vi "Mono Sample API.vi"() -> ()   [LabVIEW 2021]
uses:
  Controls/Data highway.ctl
  Controls/LED intensity Command.ctl
  Controls/State Comm.ctl
  Controls/API Command.ctl
  5323141f-2985-4b05-94d1-ece9b0648710.vi
  4ae9b108-370e-49ae-8d4b-02a5277f3aaa.vi
  <vilib>/Instr/_visa.llb/VISA Configure Serial Port (Instr).vi
panel:
  in  "offset":dbl
  in  "Comm":T1=enum."Grating Density@1"
  in  "Filter Num":i32
  in  "Refresh Button":bool
  in  "Intensity Value":i32
  out "Intensity?":bool
  in  "Intensity":bool
  out "Grating":bool
  out "Device check":bool
  in  "Device Check":bool
  in  "Set GRating Density":bool
  out "Connection?":bool
  out "error out 2":errorcluster
  out "Port out":refnum<visa-resource-name>
  out "Final response":u8
  in  "Slit":string
  out "Response":u8
  in  "error in":errorcluster
  in  "Port":refnum<visa-resource-name>
  out "Connected?":bool
  out "result":bool
  out "State":T2
  out "Wavelength":bool
  out "Shutter":bool
  out "filter":bool
  in  "Filter":bool
  in  "Shutter":bool
  in  "Wavelength(nm)":i32 min=100
  in  "Stop":bool
  out "Array":bool[](array[boolean])
  out "error out":errorcluster
  in  "error in (no error)":errorcluster
  in  "Data in out":T3={"MonoCr Port"="COM3", "Grating Selection"=enum."Grating@1", "Connection?"=TRUE, "LED Comm"=enum."LED@1", "Intensity Value"=20, "Grating Number"=1, "Wavenumber"=0, "Slit Width"=8, "Filter Num"=3, "Grating Density"=1200, "Wavelength(nm)"=532, "offset"=0.0}
  in  "Set wavelength":bool
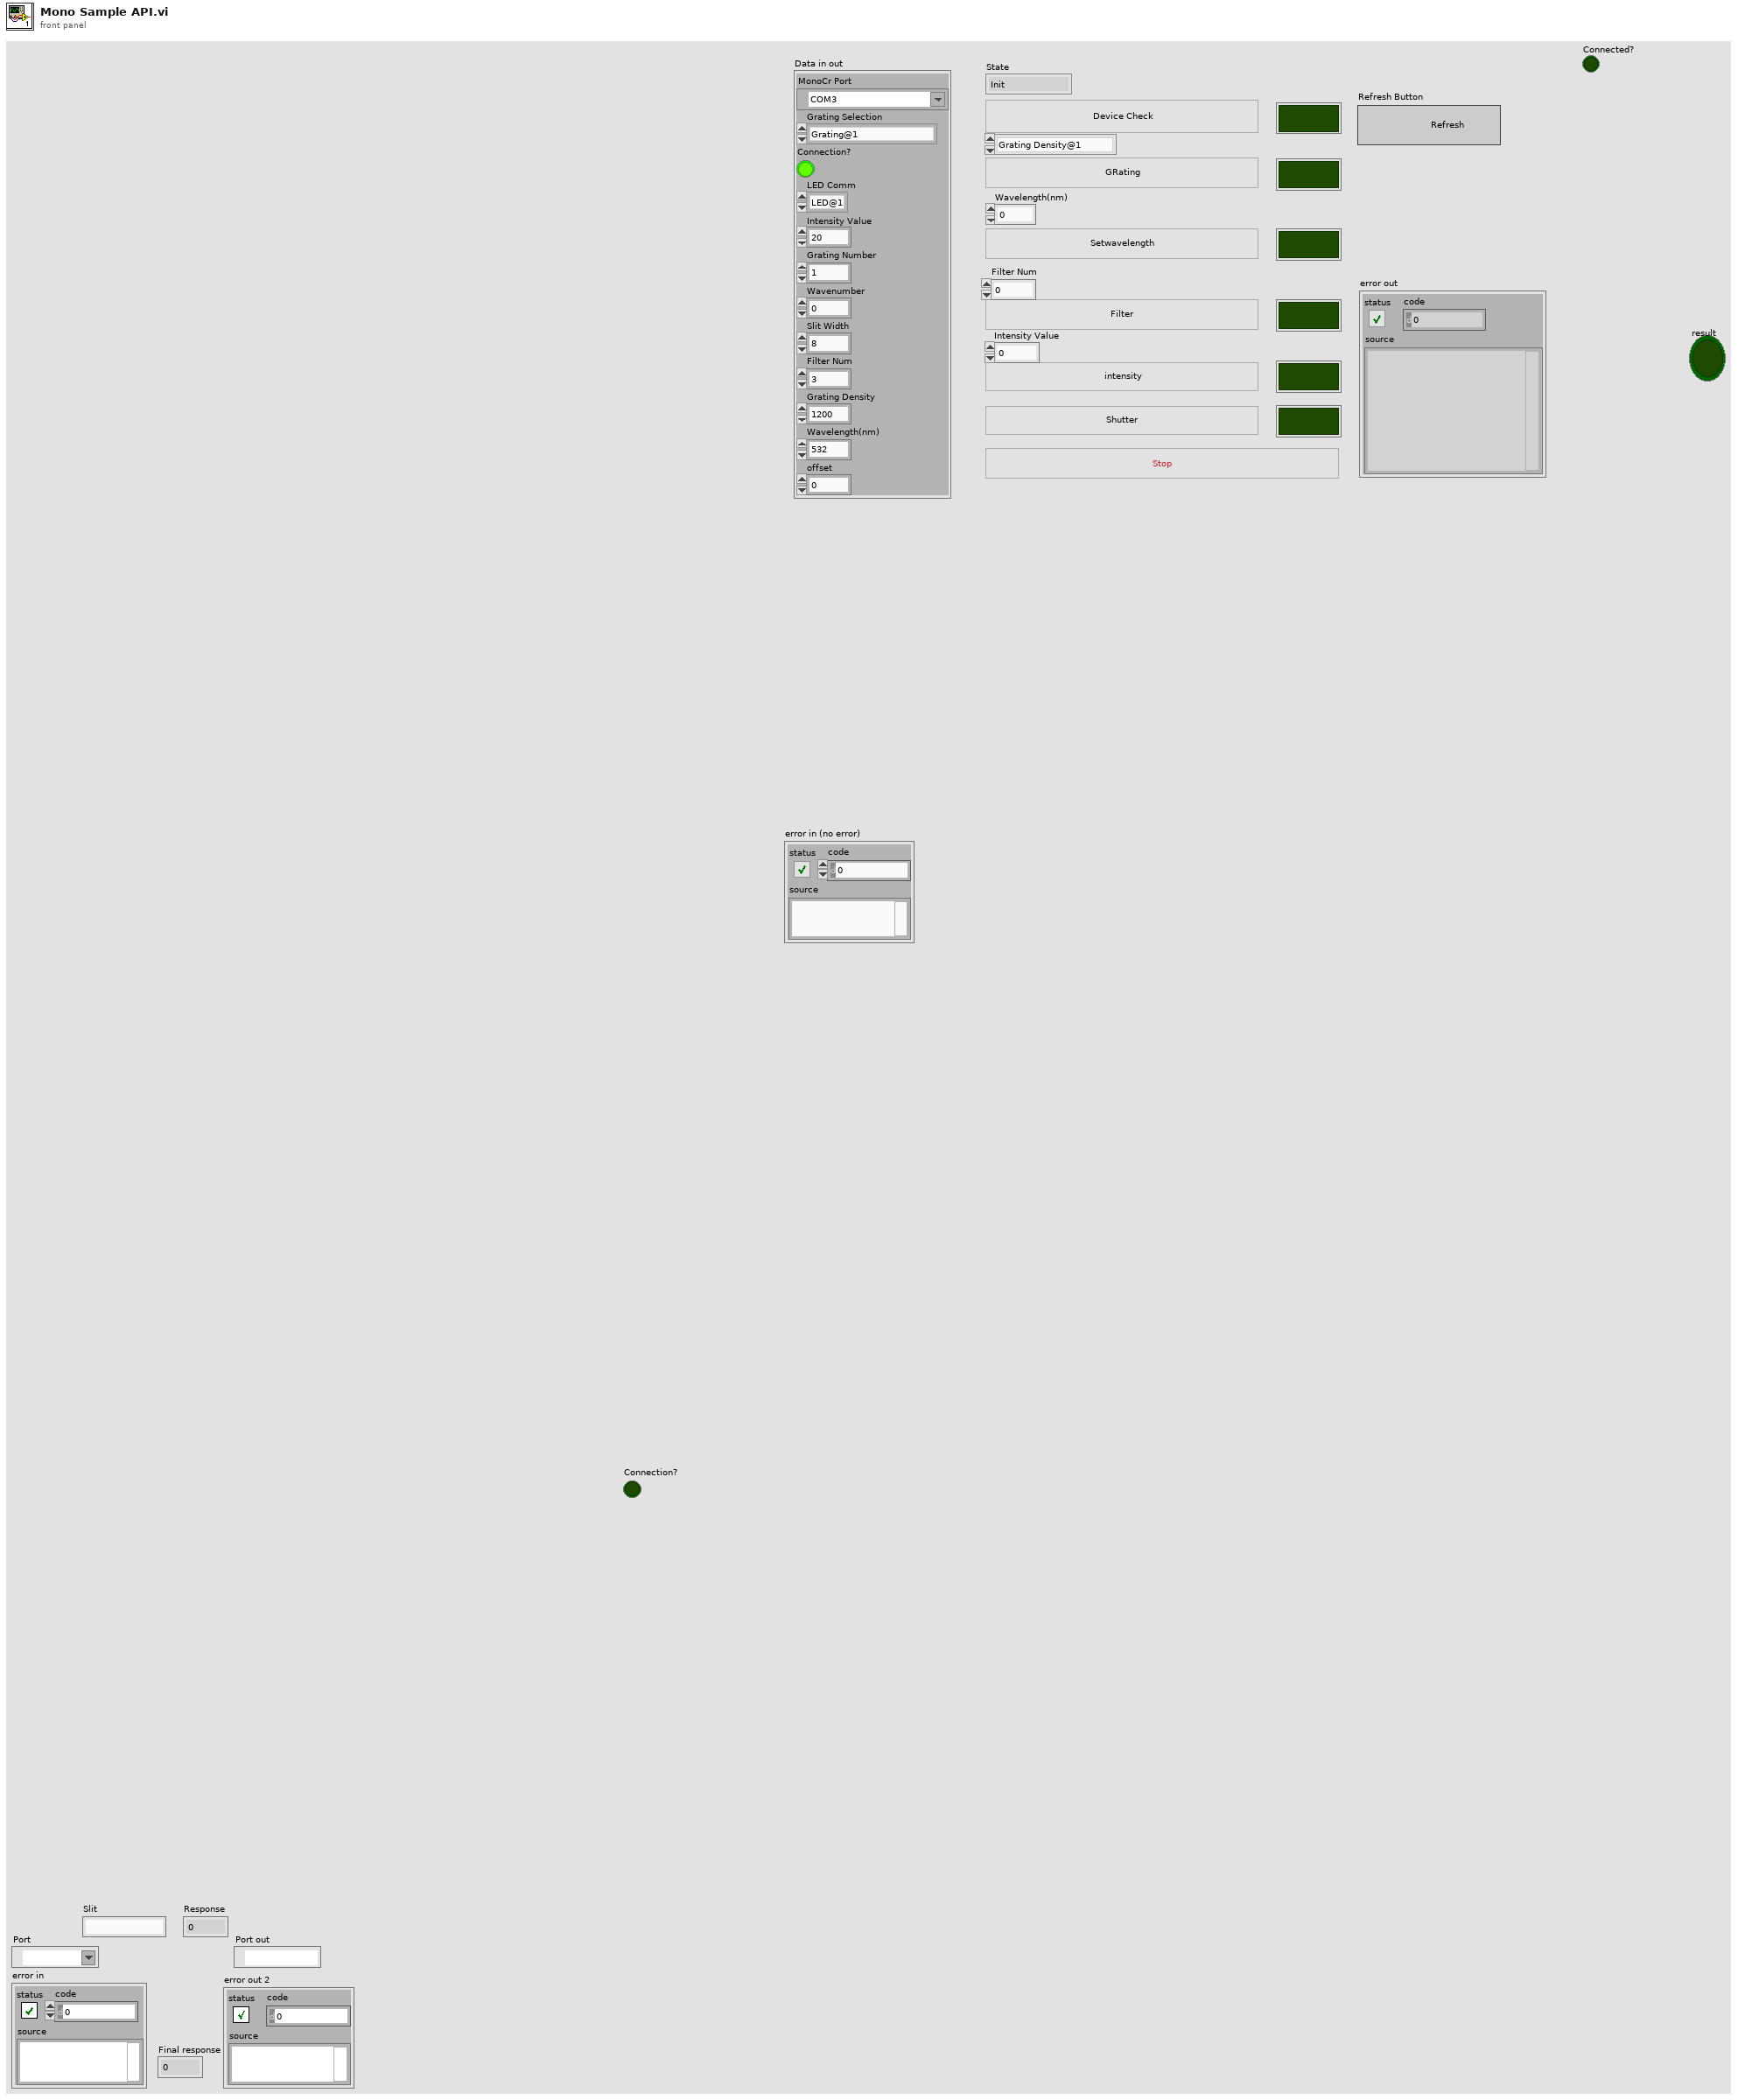
[diagram p1: front panel]
types:
  T1 = typedef "API Command.ctl" = enum16{"Init", "Device Check", "Grating Density@1", "Grating Density@2", "SetWavelength", "Filter Selection", "Shutter open", "Shutter close", "LED Intensity", "Set Grating", "Slit Width", "Stop running", "Reset Mono", "Close"}
  T2 = typedef "State Comm.ctl" = enum16{"Init", "Main", "Close"}
  T3 = typedef "Data highway.ctl" = cluster{"MonoCr Port":refnum<visa-resource-name>, "Grating Selection":enum16{"Grating@1", "Grating@2"}, "Connection?":bool, "LED Comm":T4, "Intensity Value":i32, "Grating Number":i32, "Wavenumber":i32, "Slit Width":i32, "Filter Num":i32, "Grating Density":i32, "Wavelength(nm)":i32, "offset":dbl}
  T4 = typedef "LED intensity Command.ctl" = enum16{"LED@1", "LED@2"}
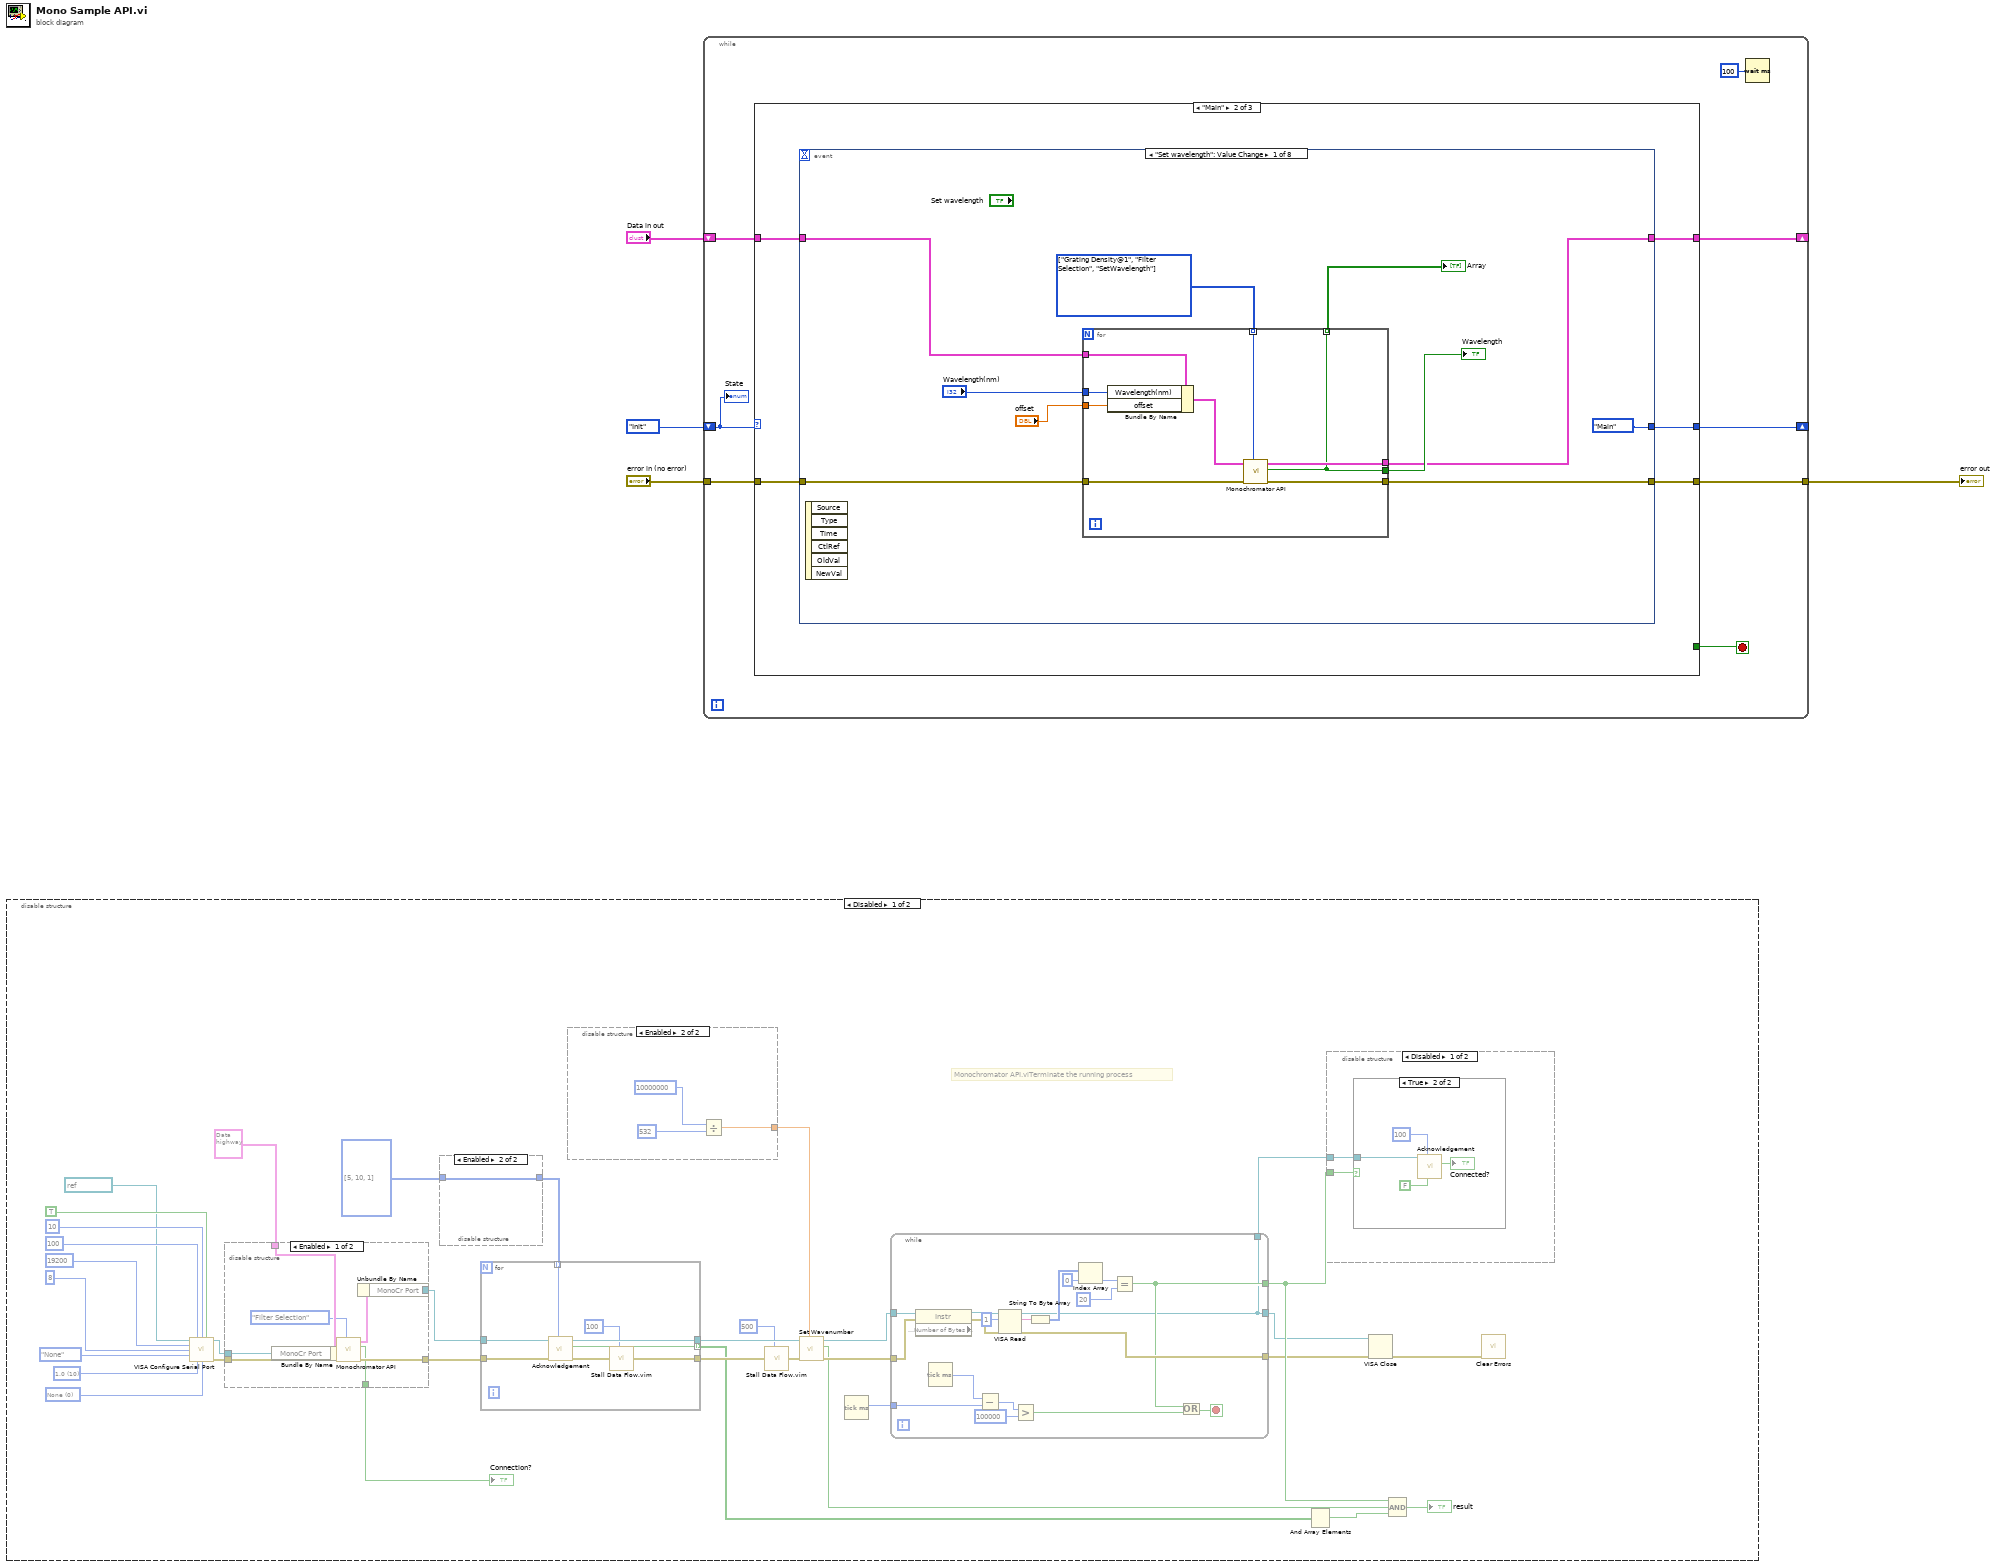
[diagram p0: block diagram]
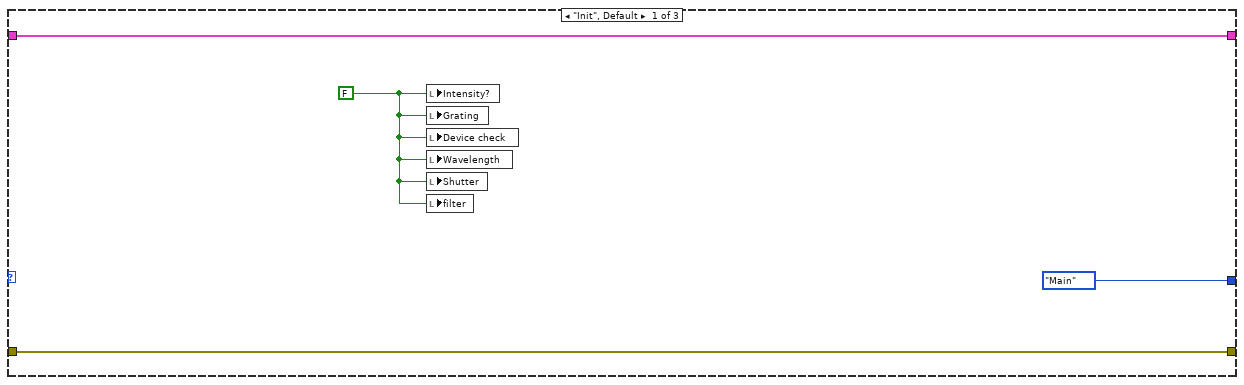
[diagram p2: hidden frame]
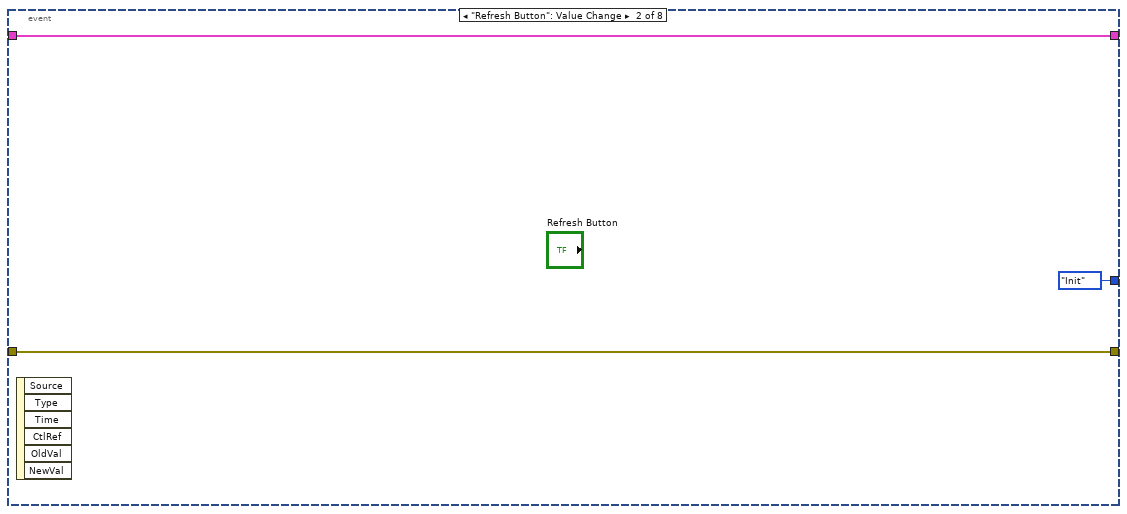
[diagram p3: hidden frame]
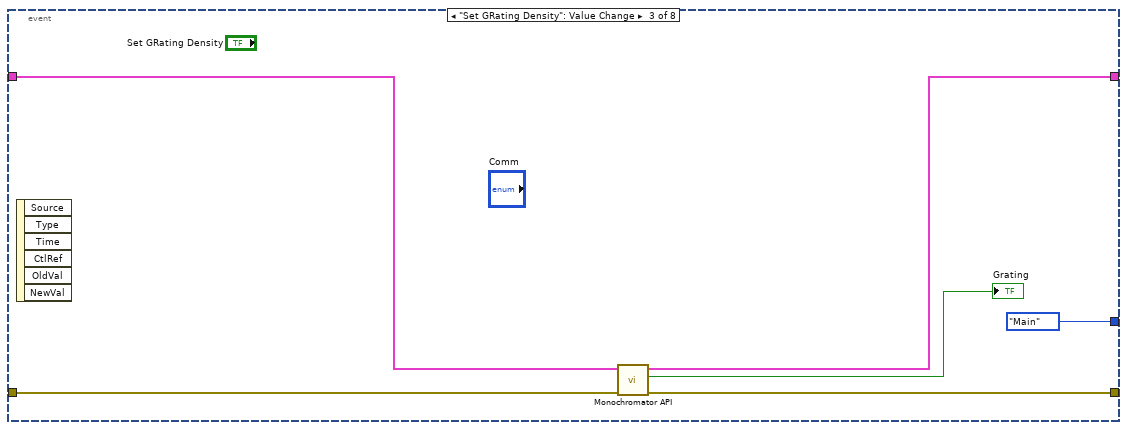
[diagram p4: hidden frame]
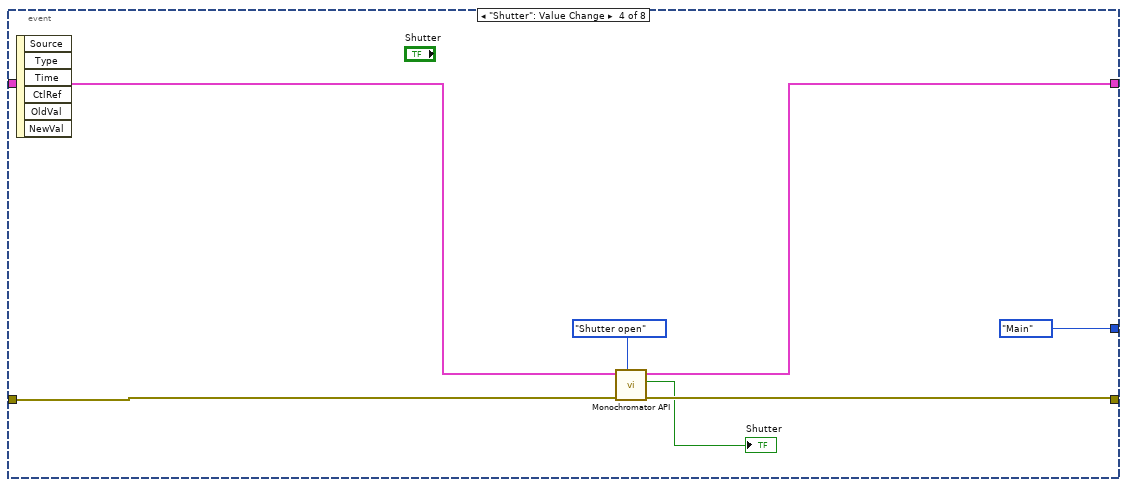
[diagram p5: hidden frame]
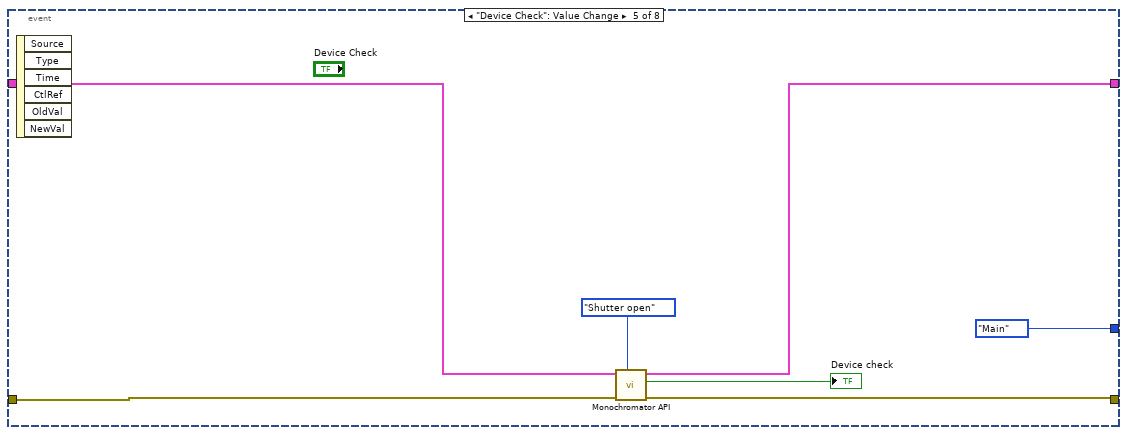
[diagram p6: hidden frame]
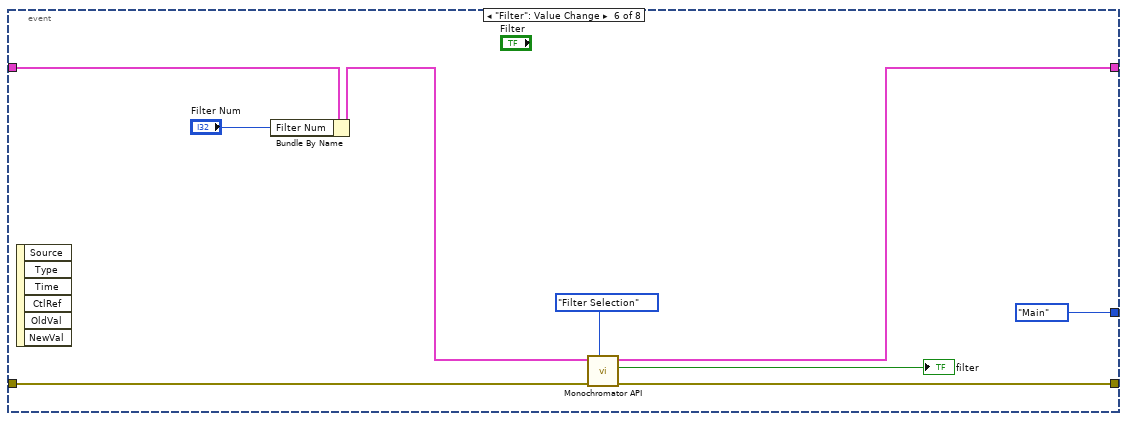
[diagram p7: hidden frame]
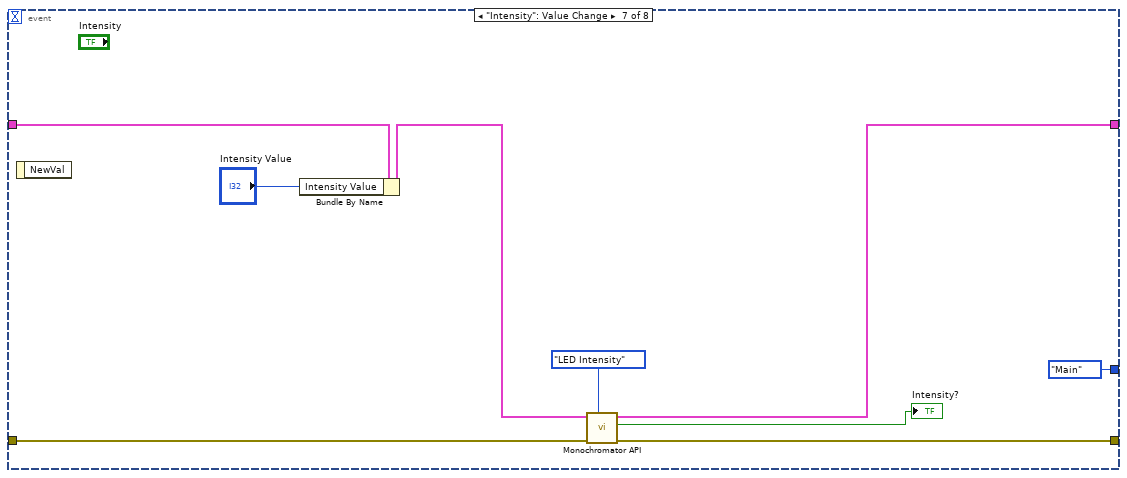
[diagram p8: hidden frame]
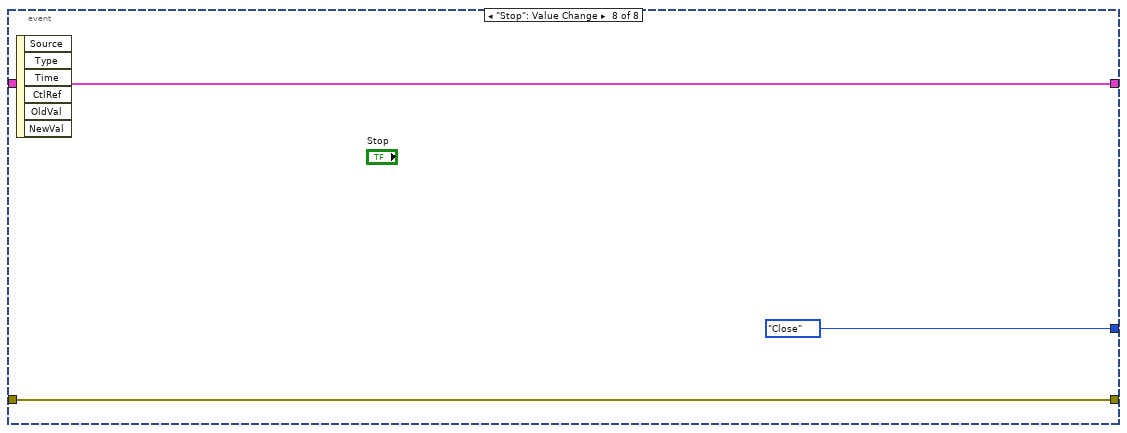
[diagram p9: hidden frame]
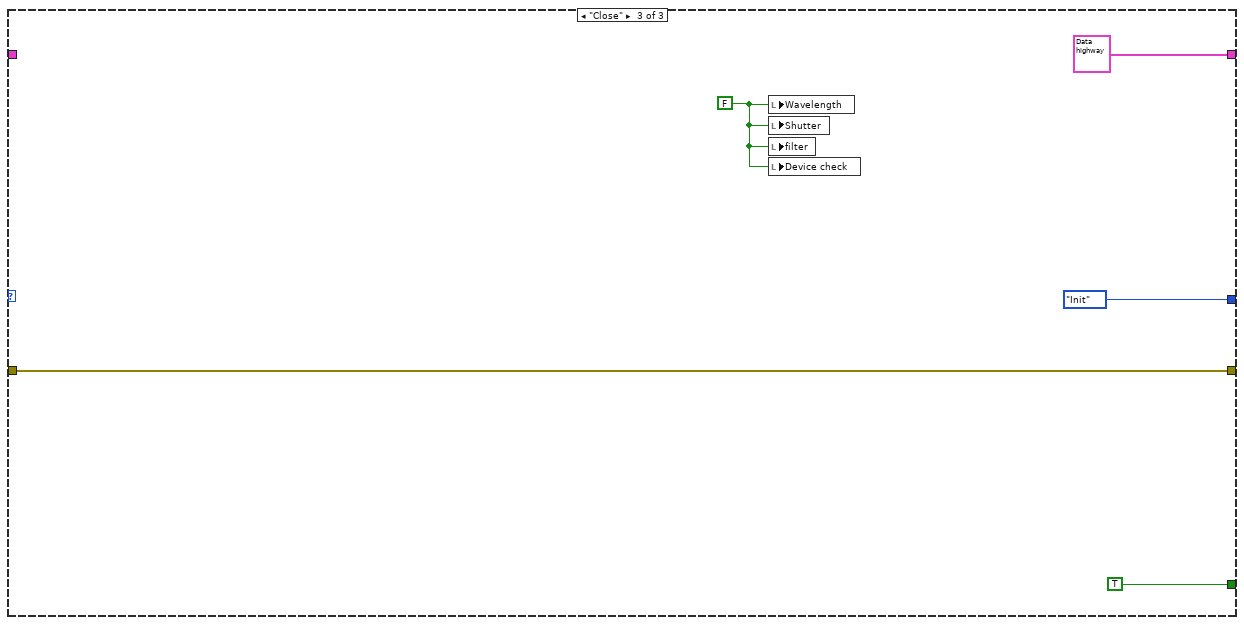
[diagram p10: hidden frame]
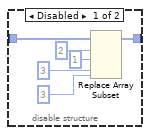
[diagram p11: hidden frame]
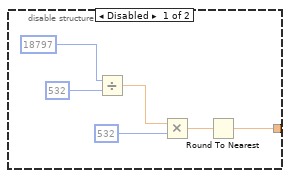
[diagram p13: hidden frame]
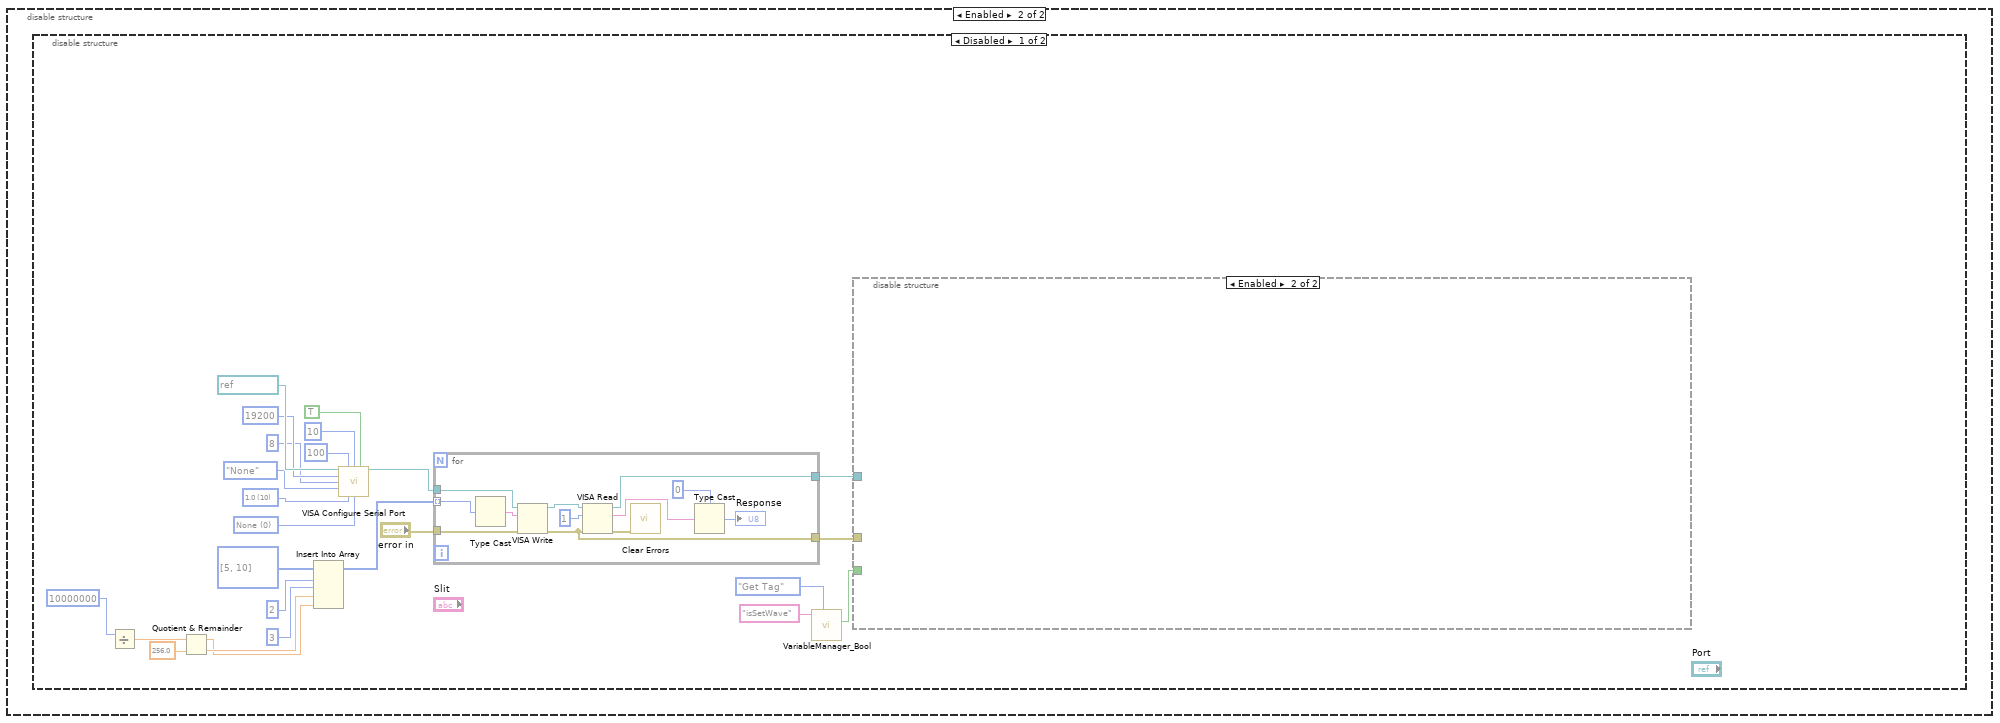
[diagram p16: hidden frame]
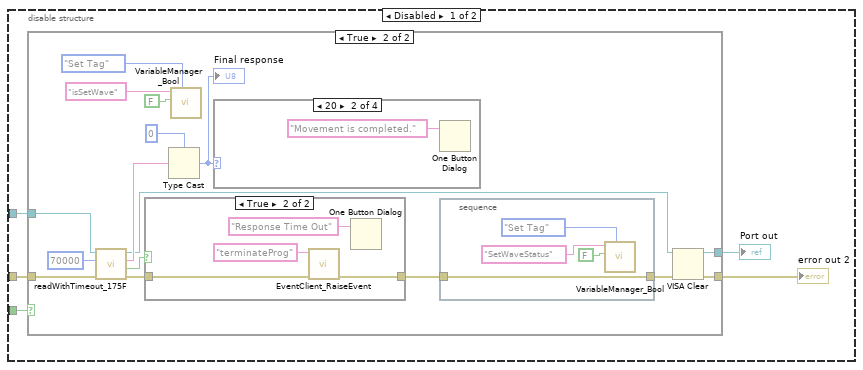
[diagram p17: hidden frame]
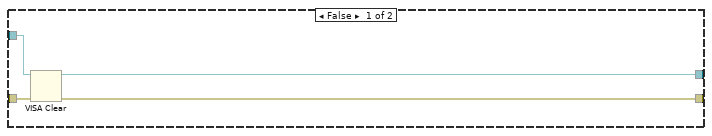
[diagram p18: hidden frame]
diagram:
  n1 = disable-structure "Diagram Disable Structure" shown="Disabled" {
    frame Disabled {
      w22 = u16 0 items=["None", "XON/XOFF", "RTS/CTS", "XON/XOFF & RTS/CTS", "DTR/DSR", "XON/XOFF & DTR/DSR"] ("flow control (0:none)")
      w23 = u16 10 items=["1.0"=10, "1.5"=15, "2.0"=20] ("stop bits (10: 1 bit)")
      # "Monochromator API.viTerminate the running process"
      n2 = call-poly "VISA Configure Serial Port"("VISA resource name"=refnum<visa-resource-name> "COM3", "timeout (10sec)"=u32 100, "termination char\n(0xA = '\\n' = LF)"=u8 10 ("termination char\n(0xA = '\\n' = LF)"), "Enable Termination\nChar (T)"=TRUE ("Enable Termination\nChar (T)"), "baud rate (9600)"=u32 19200, "data bits (8)"=u16 8, "parity (0:none)"=enum16{"None", "Odd", "Even", "Mark", "Space"}."None", "stop bits (10: 1 bit)"=w23, "flow control (0:none)"=w22) -> ("VISA resource name out"=w11:refnum<visa-resource-name>, "error out"=w14:errorcluster)  [unwired: 5 in]
      n3 = disable-structure "Diagram Disable Structure" shown="Enabled" {
        disable-tunnel: w14 -> [w54 w55]
        disable-tunnel: [w53 w55] -> w13
        disable-tunnel: T3 {"MonoCr Port"="COM3", "Grating Selection"=enum."Grating@1", "Connection?"=TRUE, "LED Comm"=enum."LED@1", "Intensity Value"=0, "Grating Number"=1, "Wavenumber"=0, "Slit Width"=8, "Filter Num"=3, "Grating Density"=0, "Wavelength(nm)"=532, "offset"=0.0} ("Data in out") -> [w52 _]
        disable-tunnel: w11 -> [w50 w56]
        disable-tunnel: [w47 w56] -> w10
        disable-tunnel: [w46 _] -> w8
        frame Enabled {
          n4 = Bundle By Name(cluster=w52, "MonoCr Port"=w50) -> (w51:T3)
          n5 = call "Monochromator API.vi"("Comm"=API_Command."Filter Selection", "error in (no error)"=w54, "Data in out"=w51) -> ("error out"=w53:errorcluster, "Connection?"=w46:bool, "Data in out"=w48:T3)  [unwired: 6 in]
          n6 = Unbundle By Name(w48) -> ("MonoCr Port"=w47:refnum<visa-resource-name>)
        }
        frame Disabled {
        }
      }
      "Connection?" <- w8
      n7 = disable-structure "Diagram Disable Structure" shown="Enabled" {
        disable-tunnel: i32[] [5, 10, 1] ("Numeric") -> [w44 w45]
        disable-tunnel: [w43 w45] -> w37
        frame Disabled {
          n8 = Replace Array Subset(array=w44, new element #1=1 ("new element/subarray"), index #1=2 ("new element/subarray"), new element #2=3 ("new element/subarray"), index #2=3 ("index")) -> (w43:i32[])
        }
        frame Enabled {
        }
      }
      n9 = for {
        tunnel: [w94] -> w20 mode=indexing
        tunnel: w13 -> [w98]
        tunnel: [w92] -> w33
        tunnel: w10 -> [w96]
        tunnel: [w95] -> w34
        tunnel: w37 -> [w93] mode=indexing
        n10 = call "Acknowledgement.vi"("Numeric"=w93, "error in (no error)"=w98, "VISA resource name"=w96) -> ("error out"=w97:errorcluster, "Connected?"=w94:bool, "VISA resource name out"=w95:refnum<visa-resource-name>)  [unwired: 6 in]
        n11 = call "Stall Data Flow.vim"("value in"=w97, "milliseconds to wait"=u32 100) -> ("value out"=w92:errorcluster)  [unwired: 1 out]
      }
      n12 = disable-structure "Diagram Disable Structure" shown="Enabled" {
        disable-tunnel: [w57 w63] -> w9
        frame Disabled {
          n13 = Divide(x=18797, y=532) -> (x/y=w60:dbl)
          n14 = Multiply(x=w60, y=532) -> (x*y=w58:dbl)
          n15 = Round To Nearest(number=w58) -> (nearest integer value=w57:dbl)
        }
        frame Enabled {
          n16 = Divide(x=10000000, y=532) -> (x/y=w63:dbl)
        }
      }
      n17 = call "Stall Data Flow.vim"("value in"=w33, "milliseconds to wait"=u32 500) -> ("value out"=w32:errorcluster)  [unwired: 1 out]
      n18 = call "Set Wavenumber.vi"("Wave number"=w9, "error in (no error)"=w32, "Comport"=w34) -> ("error out"=w35:errorcluster, "Set Success"=w18:bool, "Comport 2"=w36:refnum<visa-resource-name>)  [unwired: 6 in]
      n19 = Tick Count (ms)() -> (millisecond timer value=w30:u32)
      n20 = while {
        tunnel: w35 -> [w82]
        tunnel: [w81] -> w7
        tunnel: w36 -> [w83]
        tunnel: [w72] -> w6
        tunnel: w30 -> [w79]
        tunnel: [w74] -> w16
        tunnel: [w72] -> w15
        stop <- w76 stop-if-true
        n21 = property on="Property Node" class="Instr" props=["Serial Settings:Number of Bytes at Serial Port"](reference=w83, error in=w82) -> (reference out=w89:refnum<visa-resource-name>, error out=w90:errorcluster)  [unwired: 1 out]
        n22 = Tick Count (ms)() -> (millisecond timer value=w80:u32)
        n23 = Subtract(x=w80, y=w79) -> (x-y=w78:u32)
        n24 = VISA Read(VISA resource name=w89, byte count=u32 1, error in (no error)=w90) -> (VISA resource name out=w72:refnum<visa-resource-name>, read buffer=w86:string, error out=w81:errorcluster)  [unwired: 1 out]
        n25 = Greater?(x=w78, y=u32 100000) -> (0:w75:bool)
        n26 = String To Byte Array(string=w86) -> (unsigned byte array=w87:u8[])
        n27 = Index Array(array=w87, index=0) -> (element=w88:u8)
        n28 = Equal?(x=w88, y=u8 20) -> (x = y?=w74:bool)
        n29 = Or(x=w74, y=w75) -> (x .or. y?=w76:bool)
      }
      n30 = And Array Elements(Boolean array=w20) -> (logical AND=w19:bool)
      n31 = disable-structure "Diagram Disable Structure" shown="Disabled" {
        disable-tunnel: w16 -> [w67 _]
        disable-tunnel: w15 -> [w66 _]
        frame Disabled {
          n32 = case shown="True" w67 {
            tunnel: w66 -> [_ w71]
            frame False {
            }
            frame True {
              n33 = call "Acknowledgement.vi"("Inc"=FALSE, "Numeric"=100, "VISA resource name"=w71) -> ("Connected?"=→"Connected?":bool)  [unwired: 6 in, 2 out]
            }
          }
        }
        frame Enabled {
        }
      }
      n34 = VISA Close(VISA resource name=w6, error in (no error)=w7) -> (error out=w5:errorcluster)
      n35 = Compound Arithmetic op=AND(w16, w18, w19) -> (→"result":bool)
      n36 = call <vilib>:"Clear Errors.vi"("error in (no error)"=w5) -> ()  [unwired: 5 in, 2 out]
    }
    frame Enabled {
      n37 = disable-structure shown="Disabled" {
        frame Disabled {
          w106 = u16 0 items=["None", "XON/XOFF", "RTS/CTS", "XON/XOFF & RTS/CTS", "DTR/DSR", "XON/XOFF & DTR/DSR"] ("flow control (0:none)")
          w107 = u16 10 items=["1.0"=10, "1.5"=15, "2.0"=20] ("stop bits (10: 1 bit)")
          n38 = Divide(x=u32 10000000 ("timeOut")) -> (x/y=w116:dbl)  [unwired: 1 in]
          n39 = Quotient & Remainder(x=w116, y=256.0) -> (x-y*floor(x/y)=w118:dbl, floor(x/y)=w119:dbl)
          n40 = Insert Into Array(array=u8[] [5, 10], index=2, new element #1=u8 3 ("new element/subarray"), new element #2=w119, new element #3=w118) -> (w117:u8[])
          n41 = call-poly "VISA Configure Serial Port"("VISA resource name"=refnum<visa-resource-name> "COM3", "timeout (10sec)"=u32 100, "termination char\n(0xA = '\\n' = LF)"=u8 10 ("termination char\n(0xA = '\\n' = LF)"), "Enable Termination\nChar (T)"=TRUE ("Enable Termination\nChar (T)"), "baud rate (9600)"=u32 19200, "data bits (8)"=u16 8, "parity (0:none)"=enum16{"None", "Odd", "Even", "Mark", "Space"}."None", "stop bits (10: 1 bit)"=w107, "flow control (0:none)"=w106) -> ("VISA resource name out"=w123:refnum<visa-resource-name>)  [unwired: 5 in, 1 out]
          n42 = for {
            tunnel: w123 -> [w172]
            tunnel: "error in" -> [w171]
            tunnel: [w161] -> w122
            tunnel: [w165] -> w121
            tunnel: w117 -> [w169] mode=indexing
            n43 = Type Cast(x=w169) -> (*(type *) &x=w170:string)  [unwired: 1 in]
            n44 = VISA Write(VISA resource name=w172, write buffer=w170, error in (no error)=w171) -> (VISA resource name out=w163:refnum<visa-resource-name>, error out=w161:errorcluster)  [unwired: 1 out]
            n45 = VISA Read(VISA resource name=w163, byte count=u32 1 ("timeOut"), error in (no error)=w161) -> (VISA resource name out=w165:refnum<visa-resource-name>, read buffer=w166:string, error out=w162:errorcluster)  [unwired: 1 out]
            n46 = call <vilib>:"Clear Errors.vi"("error in (no error)"=w162) -> ()  [unwired: 5 in, 2 out]
            n47 = Type Cast(type=u8 0 ("timeOut"), x=w166) -> (*(type *) &x=→"Response":u8)
          }
          n48 = call "VariableManager_Bool.vi"("Operation"=enum16{"Get Tag", "Set Tag"}."Get Tag", "Tag"="isSetWave") -> ("Value out"=w120:bool)  [unwired: 6 in, 3 out]
          n49 = disable-structure "Diagram Disable Structure" shown="Enabled" {
            disable-tunnel: w120 -> [w128 _]
            disable-tunnel: w121 -> [w125 _]
            disable-tunnel: w122 -> [w124 _]
            frame Disabled {
              n50 = case shown="True" w128 {
                tunnel: [w132 w135] -> w127
                tunnel: [w130 w133] -> w126
                tunnel: w125 -> [w131 w140]
                tunnel: w124 -> [w129 w139]
                frame False {
                  n51 = VISA Clear(VISA resource name=w131, error in (no error)=w129) -> (VISA resource name out=w132:refnum<visa-resource-name>, error out=w130:errorcluster)
                }
                frame True {
                  n52 = call "readWithTimeout_175F.vi"("error in"=w139, "timeOut"=u32 70000, "Port"=w140) -> ("error out"=w138:errorcluster, "TimeOut"=w141:bool, "String"=w144:string, "Port out"=w136:refnum<visa-resource-name>)  [unwired: 5 in]
                  n53 = case shown="True" w141 {
                    tunnel: [w153 w155] -> w137
                    tunnel: w138 -> [w153 w154]
                    frame False {
                    }
                    frame True {
                      n54 = call "EventClient_RaiseEvent.vi"("error in (no error)"=w154, "Event"="terminateProg") -> ("error out"=w155:errorcluster)  [unwired: 9 in]
                      n55 = One Button Dialog(message="Response Time Out") -> ()  [unwired: 1 in, 1 out]
                    }
                  }
                  n56 = Type Cast(type=u8 0 ("timeOut"), x=w144) -> (*(type *) &x=w142:u8)
                  "Final response" <- w142
                  n57 = call "VariableManager_Bool.vi"("Operation"=enum16{"Get Tag", "Set Tag"}."Set Tag", "Value"=FALSE, "Tag"="isSetWave") -> ()  [unwired: 5 in, 4 out]
                  n58 = case shown="20" w142 {
                    frame 0, Default {
                    }
                    frame 20 {
                      n59 = One Button Dialog(message="Movement is completed.") -> ()  [unwired: 1 in, 1 out]
                    }
                    frame 7 {
                      n60 = One Button Dialog(message="Home limit reached.") -> ()  [unwired: 1 in, 1 out]
                    }
                    frame 14 {
                      n61 = One Button Dialog(message="Far limit reached") -> ()  [unwired: 1 in, 1 out]
                    }
                  }
                  n62 = stacked-sequence {
                    tunnel: [w152] -> w134
                    tunnel: w137 -> [w152]
                    frame #0 {
                      n63 = call "VariableManager_Bool.vi"("Operation"=enum16{"Get Tag", "Set Tag"}."Set Tag", "Value"=FALSE, "Tag"="SetWaveStatus") -> ()  [unwired: 5 in, 4 out]
                    }
                  }
                  n64 = VISA Clear(VISA resource name=w136, error in (no error)=w134) -> (VISA resource name out=w135:refnum<visa-resource-name>, error out=w133:errorcluster)
                }
              }
              "Port out" <- w127
              "error out 2" <- w126
            }
            frame Enabled {
            }
          }
        }
        frame Enabled {
        }
      }
    }
  }
  n65 = while {
    shift-right: [w179] -> _
    shift-left: State_Comm."Init" -> [w180]
    tunnel: "error in (no error)" -> [w178]
    tunnel: [w177] -> w2
    shift-right: [w175] -> _
    shift-left: "Data in out" -> [w176]
    stop <- w174 stop-if-true
    n66 = case shown="\"Main\"" w180 {
      tunnel: [State_Comm."Main" w185 State_Comm."Init"] -> w179
      tunnel: [_ _ TRUE] -> w174
      tunnel: w178 -> [w182 w189 w254]
      tunnel: [w182 w188 w254] -> w177
      tunnel: w176 -> [w183 w187 _]
      tunnel: [w183 w186 T3 {"MonoCr Port"="", "Grating Selection"=enum."Grating@1", "Connection?"=FALSE, "LED Comm"=enum."LED@1", "Intensity Value"=0, "Grating Number"=0, "Wavenumber"=0, "Slit Width"=0, "Filter Num"=0, "Grating Density"=0, "Wavelength(nm)"=0, "offset"=0.0} ("Data in out")] -> w175
      frame "Init", Default {
        w181 = FALSE ("Intensity?")
        n67 = local write "Intensity?"(w181) -> ()
        n68 = local write "Grating"(w181) -> ()
        n69 = local write "Device check"(w181) -> ()
        n70 = local write "Wavelength"(w181) -> ()
        n71 = local write "Shutter"(w181) -> ()
        n72 = local write "filter"(w181) -> ()
      }
      frame "Main" {
        n73 = event shown="[0] \"Set wavelength\": Value Change" {
          selector: _ -> [_ _ _ _ _ _ _ _]
          dyn-events: _ -> [_ _ _ _ _ _ _ _]
          timeout: _ -> [_ _ _ _ _ _ _ _]
          tunnel: w189 -> [w199 w210 w217 w220 w227 w239 w248 w250]
          tunnel: [w193 w210 w216 w219 w226 w234 w247 w250] -> w188
          tunnel: w187 -> [w198 w211 w215 w222 w229 w238 w246 w252]
          tunnel: [w191 w211 w214 w221 w228 w237 w245 w252] -> w186
          tunnel: [State_Comm."Main" State_Comm."Init" State_Comm."Main" State_Comm."Main" State_Comm."Main" State_Comm."Main" State_Comm."Main" State_Comm."Close"] -> w185
          event "Set wavelength": Value Change {
            w194 = T1[] [enum."Grating Density@1", enum."Filter Selection", enum."SetWavelength"] items=["Init", "Device Check", "Grating Density@1", "Grating Density@2", "SetWavelength", "Filter Selection", "Shutter open", "Shutter close", "LED Intensity", "Set Grating", "Slit Width", "Stop running", "Reset Mono", "Close"] ("API Comm")
            n74 = event-data() -> ()  [unwired: 1 in, 6 out]
            n75 = for {
              tunnel: w198 -> [w206]
              tunnel: [w205] -> w191
              tunnel: w199 -> [w208]
              tunnel: [w207] -> w193
              tunnel: [w202] -> w192
              tunnel: "Wavelength(nm)" -> [w203]
              tunnel: w194 -> [w201] mode=indexing
              tunnel: [w202] -> w195 mode=indexing
              tunnel: "offset" -> [w200]
              n76 = Bundle By Name(cluster=w206, "Wavelength(nm)"=w203, "offset"=w200) -> (w204:T3)
              n77 = call "Monochromator API.vi"("Comm"=w201, "error in (no error)"=w208, "Data in out"=w204) -> ("error out"=w207:errorcluster, "Connection?"=w202:bool, "Data in out"=w205:T3)  [unwired: 6 in]
            }
            "Wavelength" <- w192
            "Array" <- w195
          }
          event "Refresh Button": Value Change {
            n78 = event-data() -> ()  [unwired: 1 in, 6 out]
          }
          event "Set GRating Density": Value Change {
            n79 = event-data() -> ()  [unwired: 1 in, 6 out]
            n80 = call "Monochromator API.vi"("error in (no error)"=w217, "Data in out"=w215) -> ("error out"=w216:errorcluster, "Connection?"=→"Grating":bool, "Data in out"=w214:T3)  [unwired: 7 in]
          }
          event "Shutter": Value Change {
            n81 = event-data() -> ()  [unwired: 1 in, 6 out]
            n82 = call "Monochromator API.vi"("Comm"=API_Command."Shutter open", "error in (no error)"=w220, "Data in out"=w222) -> ("error out"=w219:errorcluster, "Connection?"=→"Shutter":bool, "Data in out"=w221:T3)  [unwired: 6 in]
          }
          event "Device Check": Value Change {
            n83 = event-data() -> ()  [unwired: 1 in, 6 out]
            n84 = call "Monochromator API.vi"("Comm"=API_Command."Shutter open", "error in (no error)"=w227, "Data in out"=w229) -> ("error out"=w226:errorcluster, "Connection?"=→"Device check":bool, "Data in out"=w228:T3)  [unwired: 6 in]
          }
          event "Filter": Value Change {
            n85 = event-data() -> ()  [unwired: 1 in, 6 out]
            n86 = Bundle By Name(cluster=w238, "Filter Num"="Filter Num") -> (w233:T3)
            n87 = call "Monochromator API.vi"("Comm"=API_Command."Filter Selection", "error in (no error)"=w239, "Data in out"=w233) -> ("error out"=w234:errorcluster, "Connection?"=→"filter":bool, "Data in out"=w237:T3)  [unwired: 6 in]
          }
          event "Intensity": Value Change {
            n88 = event-data() -> ()  [unwired: 1 in, 1 out]
            n89 = Bundle By Name(cluster=w246, "Intensity Value"="Intensity Value") -> (w242:T3)
            n90 = call "Monochromator API.vi"("Comm"=API_Command."LED Intensity", "error in (no error)"=w248, "Data in out"=w242) -> ("error out"=w247:errorcluster, "Connection?"=→"Intensity?":bool, "Data in out"=w245:T3)  [unwired: 6 in]
          }
          event "Stop": Value Change {
            n91 = event-data() -> ()  [unwired: 1 in, 6 out]
          }
        }
      }
      frame "Close" {
        w253 = FALSE ("Wavelength")
        n92 = local write "Wavelength"(w253) -> ()
        n93 = local write "Shutter"(w253) -> ()
        n94 = local write "filter"(w253) -> ()
        n95 = local write "Device check"(w253) -> ()
      }
    }
    n96 = Wait (ms)(milliseconds to wait=u32 100) -> ()  [unwired: 1 out]
    "State" <- w180
  }
  "error out" <- w2
